vi "Kugel.vi"(11 "Array (Eingang)":refnum<vi>[](array[refnum])) -> (3 "Array (Ausgang)":refnum<vi>[](array[refnum]))   [LabVIEW 2014]
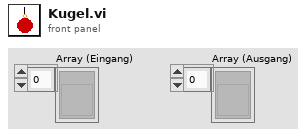
[diagram p1: front panel]
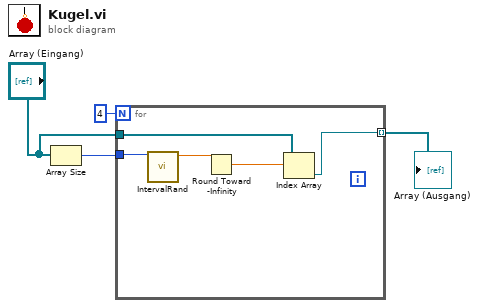
[diagram p0: block diagram]
diagram:
  n1 = Array Size(array="Array (Eingang)") -> (size(s)=w2:i32)
  n2 = for {
    N: 4 -> [_]
    tunnel: w2 -> [w9]
    tunnel: "Array (Eingang)" -> [w8]
    tunnel: [w5] -> w4 mode=indexing
    n3 = call "IntervalRand.vi"("Max"=w9) -> ("x*y"=w7:dbl)  [unwired: 10 in]
    n4 = Round Toward -Infinity(1:w7) -> (0:w6:dbl)
    n5 = Index Array(array=w8, index=w6) -> (element=w5:refnum<vi>)
  }
  "Array (Ausgang)" <- w4
